vi "Init.vi"(8 "error in (no error)":errorcluster, 11 "Instrument Driver in":refnum<class "Instrument Driver.lvclass">) -> (0 "error out":errorcluster, 1 "Post init configuration":variant, 2 "Init Result":refnum<class "Acquired Result.lvclass">, 3 "Instrument Driver out":refnum<class "Instrument Driver.lvclass">)   [LabVIEW 2019, in "Instrument Driver.lvclass"]
uses:
  Instrument Driver.lvclass
  Results/Acquired Result/Acquired Result.lvclass
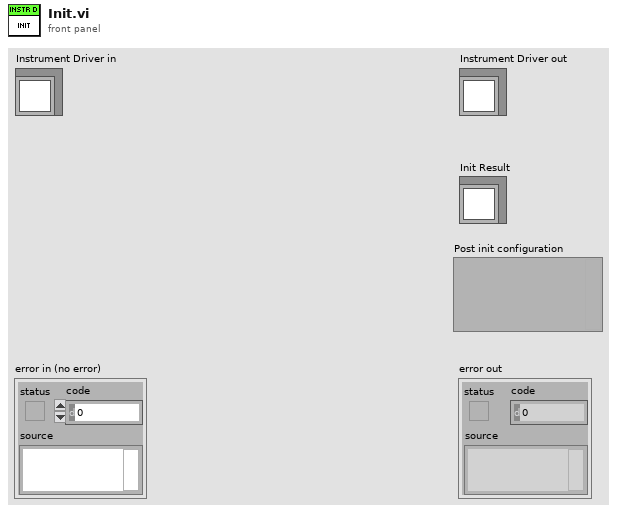
[diagram p1: front panel]
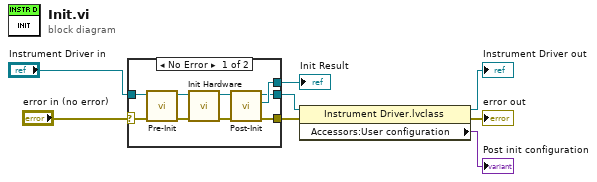
[diagram p0: block diagram]
diagram:
  n1 = case shown="No Error" "error in (no error)" {
    selector: "error in (no error)" -> [w12 w19]
    tunnel: [w10 w19] -> w4
    tunnel: [w9 w18] -> w2
    tunnel: "Instrument Driver in" -> [w13 w18]
    tunnel: [w11 _] -> w6
    frame No Error {
      n2 = call-dynamic "Pre-Init.vi"("error in (no error)"=w12, "Instrument Driver in"=w13) -> ("error out"=w15:errorcluster, "Instrument Driver out"=w17:refnum<class "Instrument Driver.lvclass">)  [unwired: 8 in]
      n3 = call-dynamic "Init Hardware.vi"("error in (no error)"=w15, "Instrument Driver in"=w17) -> ("error out"=w14:errorcluster, "Instrument Driver out"=w16:refnum<class "Instrument Driver.lvclass">)  [unwired: 8 in]
      n4 = call-dynamic "Post-Init.vi"("error in (no error)"=w14, "Instrument Driver in"=w16) -> ("error out"=w10:errorcluster, "Init Result"=w11:refnum<class "Acquired Result.lvclass">, "Instrument Driver out"=w9:refnum<class "Instrument Driver.lvclass">)  [unwired: 7 in]
    }
    frame Error {
    }
  }
  "Init Result" <- w6
  n5 = property class="Instrument Driver.lvclass"(reference=w2, error in=w4) -> (reference out=→"Instrument Driver out":refnum<class "Instrument Driver.lvclass">, error out=→"error out":errorcluster, "Accessors:User configuration"=→"Post init configuration":variant)
